vi "SaveSettings.vi"(0 "object in":refnum<class "TDMSlogg.lvclass">, 1 "Wait (s)":dbl, 2 "WFGConfig":T1={"Running"=TRUE, "Ch1"={"idxChannel"=0, "Settings out of range"=FALSE, "Carrier"={"Frequency (Hz)"=4000.0, "Amplitude (V)"=1.0, "Offset(V)"=0.0, "Symmetry(%) "=50.0, "Phase(Deg)"=0.0, "Function"=1, "Enable"=TRUE}, "Trigger"={"secRun(0=Cont)"=0.0, "secWait"=0.0, "cRepeat(0=inf)"=0, "Repeat Trigger"=FALSE, "TrigrSrc"=enum."trigrsrcNone"}, "FM Mod"={"Frequency (Hz)"=1000.0, "Amplitude (%)"=1.0, "Offset(V)"=0.0, "Symmetry(%) "=50.0, "Phase(Deg)"=0.0, "Function 2"=1, "Enable"=FALSE}}, "Ch2"={"idxChannel"=1, "Settings out of range"=FALSE, "Carrier"={"Frequency (Hz)"=1000.0, "Amplitude (V)"=1.0, "Offset(V)"=0.0, "Symmetry(%) "=50.0, "Phase(Deg)"=0.0, "Function"=1, "Enable"=FALSE}, "Trigger"={"secRun(0=Cont)"=0.0, "secWait"=0.0, "cRepeat(0=inf)"=0, "Repeat Trigger"=FALSE, "TrigrSrc"=enum."trigrsrcNone"}, "FM Mod"={"Frequency (Hz)"=1000.0, "Amplitude (%)"=1.0, "Offset(V)"=0.0, "Symmetry(%) "=50.0, "Phase(Deg)"=0.0, "Function 2"=1, "Enable"=FALSE}}, "SyncronizeState"=enum."Independent"} {"Ch2"."FM Mod"."Function 2" items=["DC"=0, "Sine"=1, "Square"=2, "Triangle"=3, "RampUp"=4, "RampDown"=5, "Noise"=6, "Pulse"=7, "Custom"=30]; "Ch2"."Carrier"."Function" items=["DC"=0, "Sine"=1, "Square"=2, "Triangle"=3, "RampUp"=4, "RampDown"=5, "Noise"=6, "Pulse"=7, "Custom"=30]; "Ch1"."FM Mod"."Function 2" items=["DC"=0, "Sine"=1, "Square"=2, "Triangle"=3, "RampUp"=4, "RampDown"=5, "Noise"=6, "Pulse"=7, "Custom"=30]; "Ch1"."Carrier"."Function" items=["DC"=0, "Sine"=1, "Square"=2, "Triangle"=3, "RampUp"=4, "RampDown"=5, "Noise"=6, "Pulse"=7, "Custom"=30]}, 3 "ThresholdRange":cluster{"Lower value":sgl, "Upper value":sgl}={"Lower value"=128.0, "Upper value"=255.0} {"Upper value" format="%.2f"; "Lower value" format="%.2f"}, 4 "current time":timestamp, 5 "error in (no error)":errorcluster) -> (14 "object out":refnum<class "TDMSlogg.lvclass">, 19 "error out":errorcluster)   [LabVIEW 2019, in "TDMSlogg.lvclass"]
uses:
  TDMSlogg.lvclass
  AD2_WFG_SDK_class/AD2TriggerSources.ctl
  AD2_SDK_class/AD2_SDK.lvclass
  AD2_WFG_SDK_class/WFGCh.ctl
  AD2_WFG_SDK_class/AD2_WFG_SDK.lvclass
  AD2_WFG_SDK_class/WFG.ctl
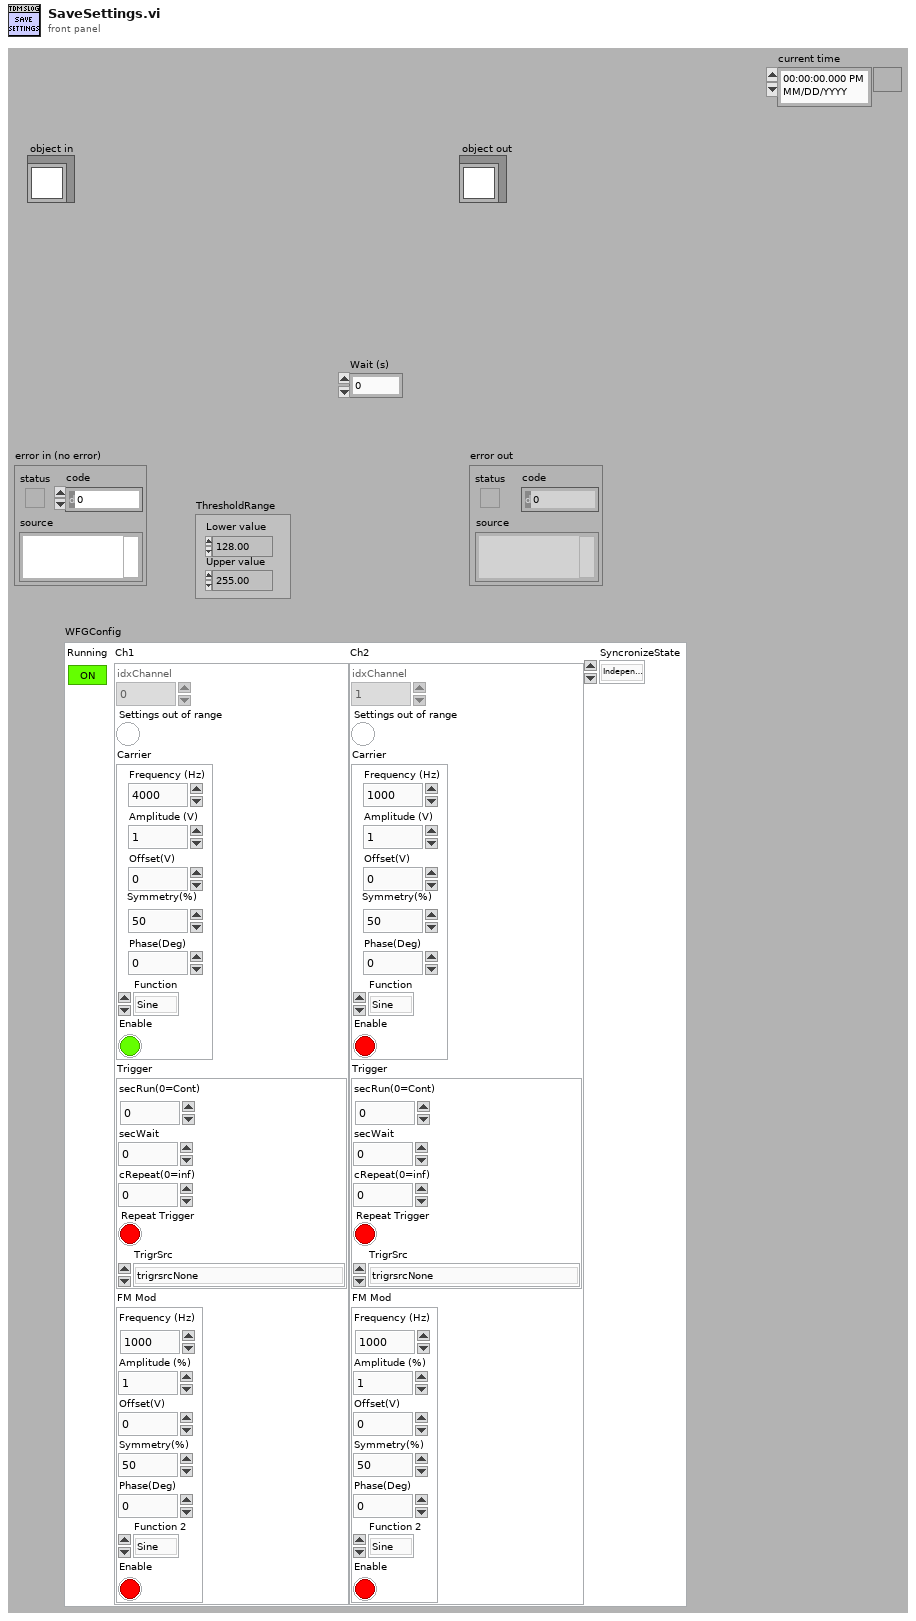
[diagram p1: front panel]
types:
  T1 = typedef "AD2_WFG_SDK.lvclass/WFG.ctl" = cluster{"Running":bool, "Ch1":T2, "Ch2":T2, "SyncronizeState":enum16{"Independent", "Ch1Master", "Ch2Master"}}
  T2 = typedef "AD2_WFG_SDK.lvclass/WFGCh.ctl" = cluster{"idxChannel":i32, "Settings out of range":bool, "Carrier":cluster{"Frequency (Hz)":dbl, "Amplitude (V)":dbl, "Offset(V)":dbl, "Symmetry(%) ":dbl, "Phase(Deg)":dbl, "Function":u16, "Enable":bool}, "Trigger":cluster{"secRun(0=Cont)":dbl, "secWait":dbl, "cRepeat(0=inf)":i32, "Repeat Trigger":bool, "TrigrSrc":T3}, "FM Mod":cluster{"Frequency (Hz)":dbl, "Amplitude (%)":dbl, "Offset(V)":dbl, "Symmetry(%) ":dbl, "Phase(Deg)":dbl, "Function 2":u16, "Enable":bool}}
  T3 = typedef "AD2_SDK.lvclass/AD2TriggerSources.ctl" = enum8{"trigrsrcNone", "trigsrcPC", "trigsrcDetectorAnalogIn", "trigsrcDetectorDigitalIn", "trigsrcAnalogIn", "trigsrcDigitalIn", "trigsrcDigitalOut", "trigsrcAnalogOut1", "trigsrcAnalogOut2", "trigsrcAnalogOut3", "trigsrcAnalogOut4", "trigsrcExternal1", "trigsrcExternal2", "trigsrcExternal3", "trigsrcExternal4", ""}
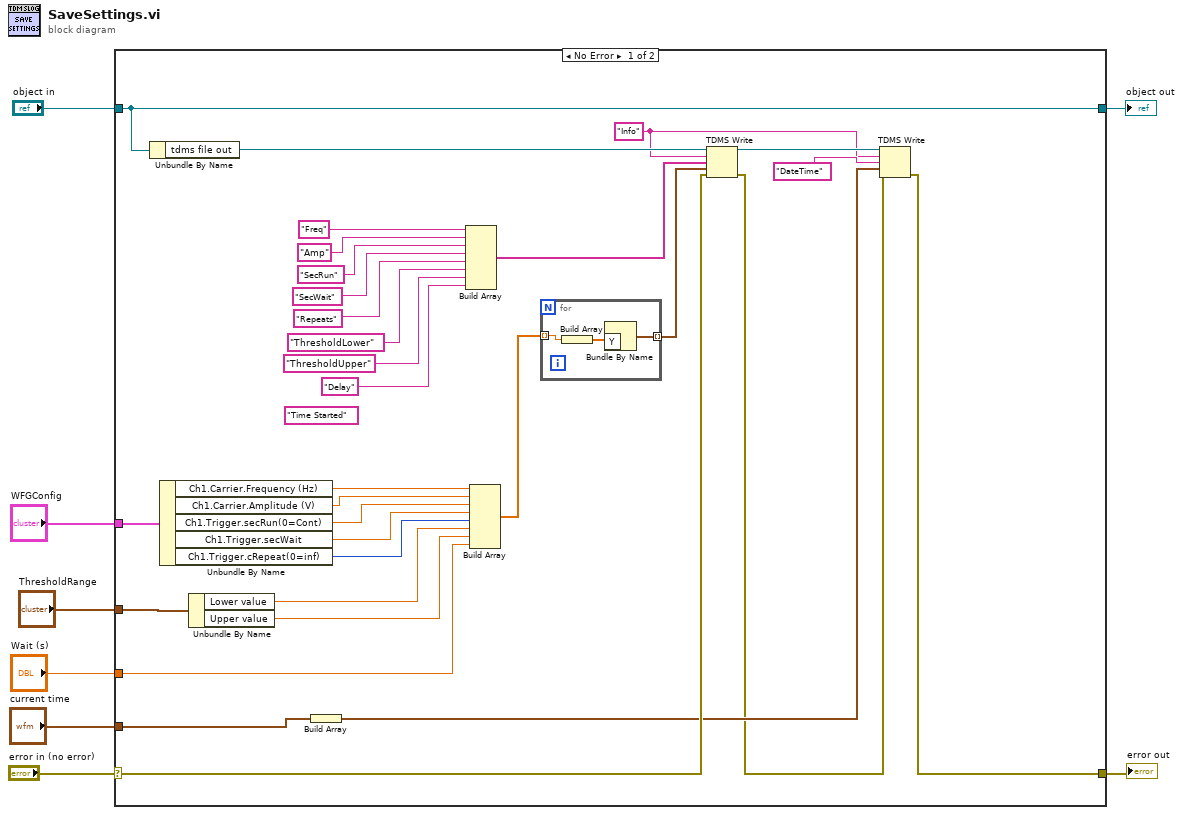
[diagram p0: block diagram]
diagram:
  n1 = case shown="No Error" "error in (no error)" {
    selector: "error in (no error)" -> [w25 w44]
    tunnel: [w9 w44] -> w7
    tunnel: [w39 w43] -> w5
    tunnel: "object in" -> [w39 w43]
    tunnel: "WFGConfig" -> [w38 _]
    tunnel: "ThresholdRange" -> [w22 _]
    tunnel: "Wait (s)" -> [w16 _]
    tunnel: "current time" -> [w11 _]
    frame No Error {
      (unwired) "Time Started" ("element")
      w12 = "Info" ("group name in (Untitled)")
      n2 = Unbundle By Name(w39) -> ("tdms file out"=w26:refnum<k34>)
      n3 = Unbundle By Name(w38) -> ("Ch1.Carrier.Frequency (Hz)"=w32:dbl, "Ch1.Carrier.Amplitude (V)"=w31:dbl, "Ch1.Trigger.secRun(0=Cont)"=w30:dbl, "Ch1.Trigger.secWait"=w29:dbl, "Ch1.Trigger.cRepeat(0=inf)"=w28:i32)
      n4 = Unbundle By Name(w22) -> ("Lower value"=w21:sgl, "Upper value"=w20:sgl)
      n5 = Build Array(w11) -> (w14:timestamp[])
      n6 = Build Array("Freq", "Amp", "SecRun", "SecWait", "Repeats", "ThresholdLower", "ThresholdUpper", "Delay" ("element")) -> (w27:string[])
      n7 = Build Array(w32, w31, w30, w29, w28, w21, w20, w16) -> (w24:dbl[])
      n8 = for {
        tunnel: w24 -> [w42] mode=indexing
        tunnel: [w40] -> w23 mode=indexing
        n9 = Build Array(w42) -> (w41:dbl[])
        n10 = Bundle By Name("Y"=w41) -> (w40:waveform(dbl))  [unwired: 1 in]
      }
      n11 = TDMS Write(0:w26, 5:w12, 7:w27, 9:w23, 11:w25) -> (4:w15:refnum<k34>, 15:w10:errorcluster)  [unwired: 1 in, 2 out]
      n12 = TDMS Write(0:w15, 5:w12, 7:"DateTime" ("group name in (Untitled)"), 9:w14, 11:w10) -> (15:w9:errorcluster)  [unwired: 1 in, 3 out]
    }
    frame Error {
    }
  }
  "error out" <- w7
  "object out" <- w5
